vi "Launch.vi"(8 "error in":errorcluster) -> (0 "error out":errorcluster, 3 "SplashScreen":T1)   [LabVIEW 2013, in "configuration library.lvlib" / "splash screen.lvlib"]
uses:
  splash screen.lvlib
  splash screen.ctl
  notifier data.ctl
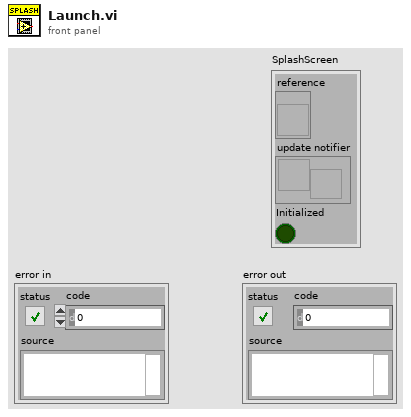
[diagram p1: front panel]
types:
  T1 = typedef "configuration library.lvlib/splash screen.lvlib/splash screen.ctl" = cluster{"reference":refnum<vi>, "update notifier":refnum<notifier>, "Initialized":bool}
  T2 = typedef "configuration library.lvlib/splash screen.lvlib/notifier data.ctl" = cluster{"Text":string, "percent":dbl}
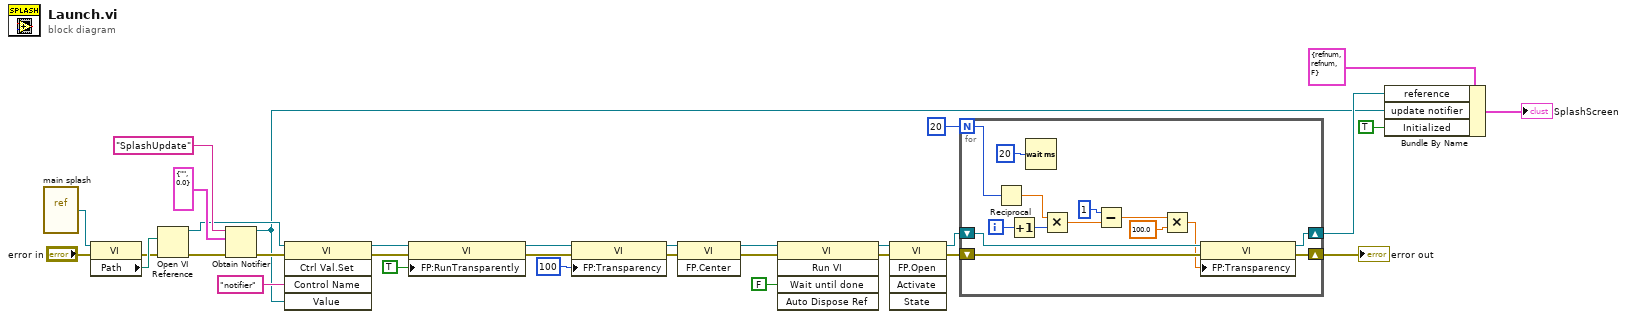
[diagram p0: block diagram]
diagram:
  n1 = vi-ref "main splash.vi"() -> (w8:refnum<vi>)
  n2 = property class="VI"(reference=w8, error in="error in") -> (error out=w4:errorcluster, "Path"=w7:path)  [unwired: 1 out]
  n3 = Open VI Reference(vi path=w7, error in (no error)=w4) -> (vi reference=w6:refnum<vi>, error out=w3:errorcluster)  [unwired: 4 in]
  n4 = Obtain Notifier(name (unnamed)="SplashUpdate" ("Notifier Name"), notification data type=T2 {"Text"="", "percent"=0.0} ("Update"), error in (no error)=w3) -> (notifier out=w1:refnum<notifier>, error out=w18:errorcluster)  [unwired: 1 in, 1 out]
  n5 = invoke class="VI" method="Ctrl Val.Set"(reference=w6, error in=w18, "Control Name"="notifier", "Value"=w1) -> (reference out=w15:refnum<vi>, error out=w14:errorcluster)  [unwired: 1 in, 3 out]
  n6 = property class="VI"(reference=w15, error in=w14, "FP:RunTransparently"=TRUE ("Front Panel Window:Run VI Transparently")) -> (reference out=w27:refnum<vi>, error out=w26:errorcluster)
  n7 = property class="VI"(reference=w27, error in=w26, "FP:Transparency"=u8 100 ("Front Panel Window:Transparency")) -> (reference out=w23:refnum<vi>, error out=w24:errorcluster)
  n8 = invoke class="VI" method="FP.Center"(reference=w23, error in=w24) -> (reference out=w30:refnum<vi>, error out=w29:errorcluster)  [unwired: 1 in, 1 out]
  n9 = invoke class="VI" method="Run VI"(reference=w30, error in=w29, "Wait until done"=FALSE ("Wait Until Done")) -> (reference out=w22:refnum<vi>, error out=w21:errorcluster)  [unwired: 2 in, 3 out]
  n10 = invoke class="VI" method="FP.Open"(reference=w22, error in=w21) -> (reference out=w20:refnum<vi>, error out=w19:errorcluster)  [unwired: 3 in, 3 out]
  n11 = for {
    N: 20 -> [w40]
    shift-right: [w43] -> w10
    shift-left: w20 -> [w45]
    shift-right: [w46] -> w12
    shift-left: w19 -> [w44]
    i -> [w34]
    n12 = Reciprocal(x=w40) -> (1/x=w36:dbl)
    n13 = Increment(x=w34) -> (x+1=w33:i32)
    n14 = Wait (ms)(milliseconds to wait=u32 20) -> ()  [unwired: 1 out]
    n15 = Multiply(x=w36, y=w33) -> (x*y=w35:dbl)
    n16 = Subtract(x=1, y=w35) -> (x-y=w39:dbl)
    n17 = Multiply(x=w39, y=100.0) -> (x*y=w37:dbl)
    n18 = property class="VI"(reference=w45, error in=w44, "FP:Transparency"=w37) -> (reference out=w43:refnum<vi>, error out=w46:errorcluster)
  }
  "error out" <- w12
  n19 = Bundle By Name(cluster=T1 {"reference"=refnum, "update notifier"=refnum, "Initialized"=FALSE} ("SplashScreen"), "reference"=w10, "update notifier"=w1, "Initialized"=TRUE ("Show Splash Screen")) -> (→"SplashScreen":T1)
